vi "QPalette.vi"(8 "Error In":errorcluster, 10 "button":u32(colorbox)) -> (0 "Error Out":errorcluster, 3 "New QPalette":refnum<class "QPalette.lvclass">)   [LabVIEW 2014, in "QPalette.lvclass"]
doc: "LabVIEW-specific documentation is not yet available. See <b>https://doc.qt.io/qt-5/qpalette.html#QPalette</b>"
uses:
  QPalette.lvclass
  LQ Core/LQSerialData/LQSerialData.lvclass/LQSerialData.ctl
  LQ Core/LQ Core.lvlib
  LQ Core/LQSerialData/LQSerialData.lvclass
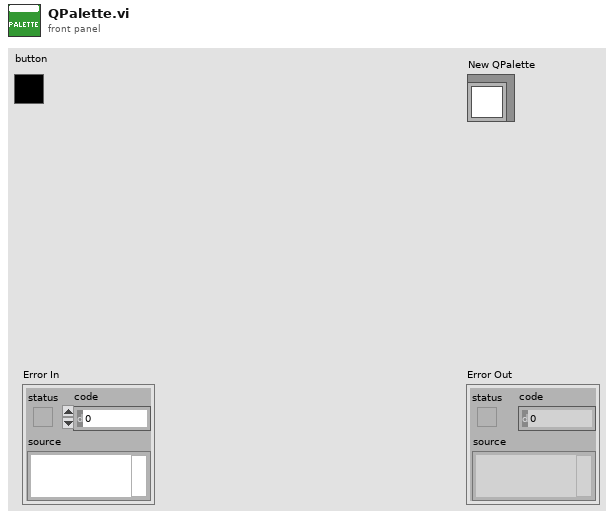
[diagram p1: front panel]
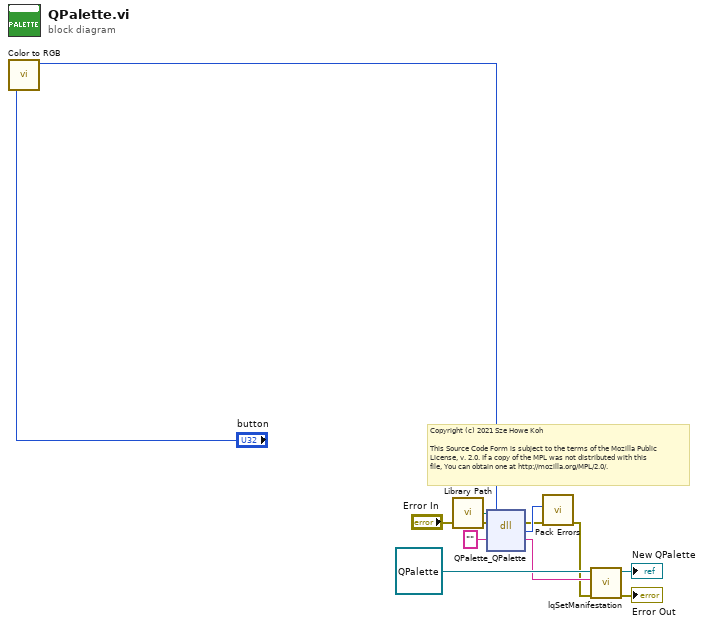
[diagram p0: block diagram]
diagram:
  # "Copyright (c) 2021 Sze Howe Koh\n\nThis Source Code Form is subject to the terms of the Mozilla Public\nLicense, v. 2.0. If a copy of the MPL was not distributed with this\nfile, You can obtain one at http://mozilla.org/MPL/2.0/."
  n1 = call <vilib>:"Color to RGB.vi"("Color"="button") -> ("Resolved Color"=w1:u32)  [unwired: 3 out]
  n2 = call "Library Path.vi"() -> ("Library Path"=w7:path)
  n3 = dll-call lib="?" fn="QPalette_QPalette"(path in=w7, error in="Error In", "_retVal"="", "button"=w1) -> (error out=w5:errorcluster, w6:i32, "_retVal"=w8:string)  [unwired: 2 in, 1 out]
  n4 = call "Pack Errors.vi"("Error In"=w5, "Error Code"=w6) -> ("Error Out"=w4:errorcluster)  [unwired: 9 in]
  n5 = call "lqSetManifestation.vi"("Error In"=w4, "Manifestation"=w8, "LQSerialData in"=refnum<class "QPalette.lvclass"> refnum ("QPalette")) -> ("Error Out"=→"Error Out":errorcluster, "LQSerialData out"=→"New QPalette":refnum<class "QPalette.lvclass">)  [unwired: 7 in]
